vi "HAL camera set temp.vi"(1 "Temp. Set Point":i32) -> (0 "error out":errorcluster)   [LabVIEW 2011]
uses:
  ATMCD32D.DLL
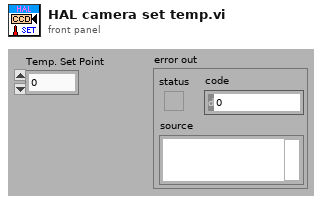
[diagram p1: front panel]
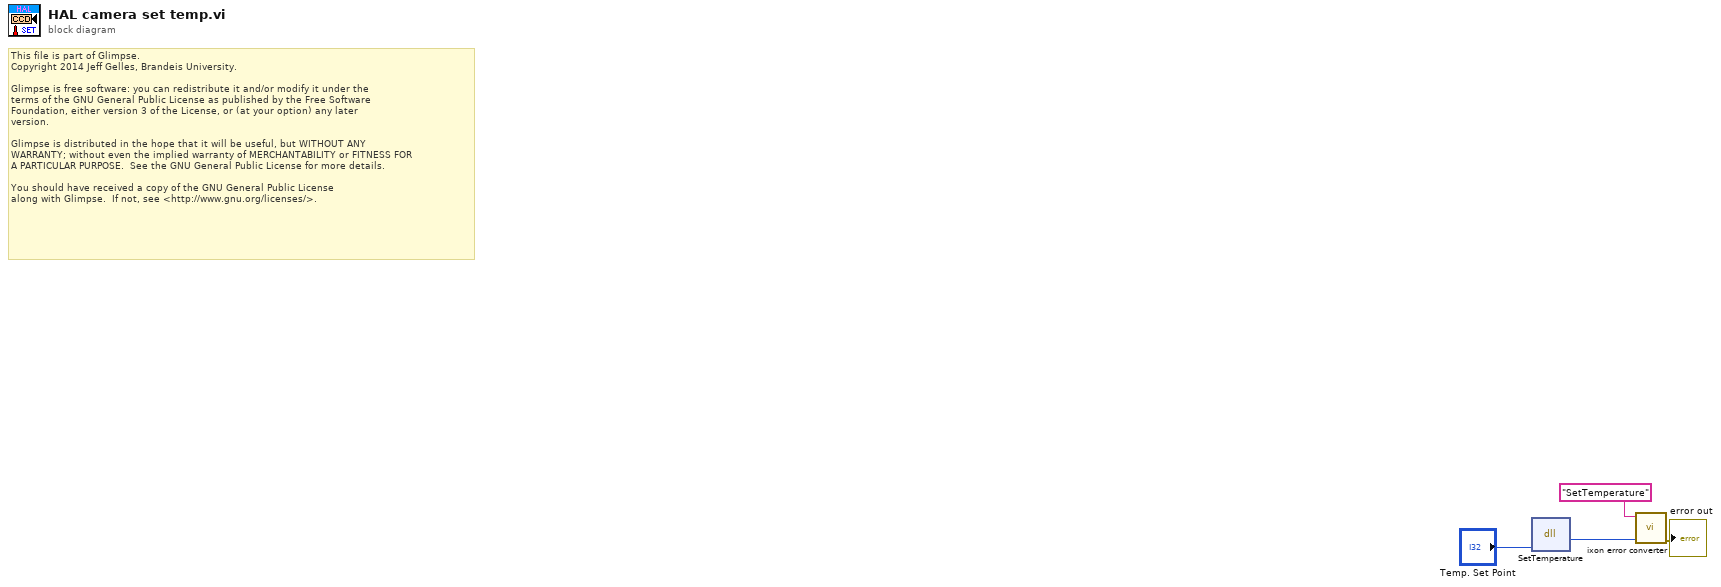
[diagram p0: block diagram]
diagram:
  # "This file is part of Glimpse. \nCopyright 2014 Jeff Gelles, Brandeis University.    \n\nGlimpse is free software: you can redistribute it and/or modify it under the \nterms of the GNU General Public License as published by the Free Software \nFoundation, either version 3 of the License, or (at your option) any later \nversion.\n\nGlimpse is distributed in the hope that it will be useful, but WITHOUT ANY \nWARRANTY; without even the implied warranty of MERCHANTABILITY or FITNESS FOR \nA PARTICULAR PURPOSE.  See the GNU General Public License for more details.\n\nYou should have received a copy of the GNU General Public License\nalong with Glimpse.  If not, see <http://www.gnu.org/licenses/>."
  n1 = dll-call lib="ATMCD32D.DLL" fn="SetTemperature"("Temp. Set Point") -> (w3:u32)  [unwired: 4 in, 2 out]
  n2 = call "ixon error converter.vi"("Andor error code"=w3, "source"="SetTemperature") -> ("error out"=→"error out":errorcluster)  [unwired: 5 out]
